vi "Simulated_Field_Read_Field_List.vi"() -> (0 "error out":errorcluster, 3 "section names":string[](array[string]))   [LabVIEW 2019, in "Simulated_Field.lvlib"]
uses:
  Simulated_Field.lvlib
  <vilib>/Utility/config.llb/NI_LVConfig.lvlib
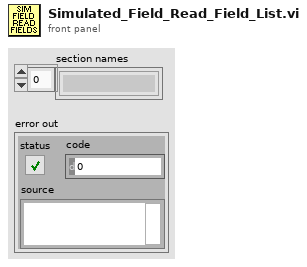
[diagram p1: front panel]
types:
  T1 = typedef "NI_LVConfig.lvlib/Config Data RefNum.ctl" = refnum<k1>
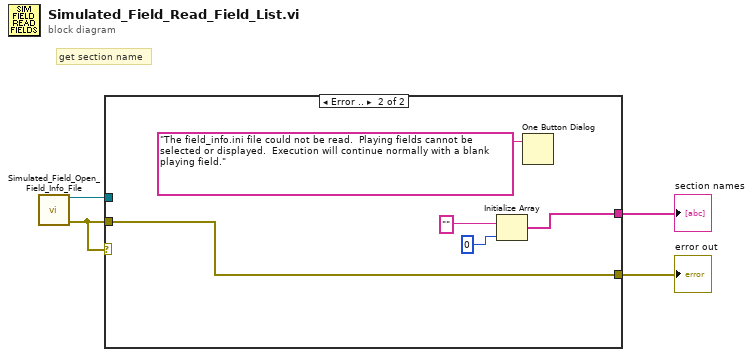
[diagram p0: block diagram]
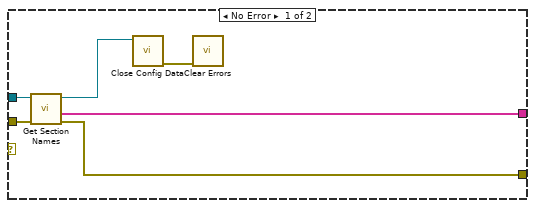
[diagram p2: hidden frame]
diagram:
  # "get section name"
  n1 = call "Simulated_Field_Open_Field_Info_File.vi"() -> ("error out"=w1:errorcluster, "Refnum out"=w2:T1)  [unwired: 10 in]
  n2 = case shown="Error .." w1 {
    tunnel: [w9 w15] -> w4
    tunnel: w1 -> [w8 w15]
    tunnel: [w7 w11] -> w3
    tunnel: w2 -> [w6 _]
    frame No Error {
      n3 = call <vilib>:"Get Section Names.vi"("error in (no error)"=w8, "refnum"=w6) -> ("error out"=w9:errorcluster, "section names"=w7:string[], "refnum out"=w10:T1)  [unwired: 7 in]
      n4 = call <vilib>:"Close Config Data.vi"("refnum"=w10) -> ("error out"=w5:errorcluster)  [unwired: 9 in, 1 out]
      n5 = call <vilib>:"Clear Errors.vi"("error in (no error)"=w5) -> ()  [unwired: 5 in, 2 out]
    }
    frame Error {
      n6 = Initialize Array("" ("String"), 0 ("dimension size")) -> (w11:string[])
      n7 = One Button Dialog(message="The field_info.ini file could not be read.  Playing fields cannot be selected or displayed.  Execution will continue normally with a blank playing field.") -> ()  [unwired: 1 in, 1 out]
    }
  }
  "error out" <- w4
  "section names" <- w3
